vi "FollowAttackerTactic.vi"(8 "error in (no error)":errorcluster, 9 "Game in":refnum<class "Game.lvclass">, 10 "Robot":refnum<class "Robot.lvclass">, 11 "FollowAttackerTactic in":refnum<class "FollowAttackerTactic.lvclass">) -> (0 "error out":errorcluster, 2 "Robot out":refnum<class "Robot.lvclass">, 3 "FollowAttackerTactic out":refnum<class "FollowAttackerTactic.lvclass">)   [LabVIEW 2018, in "FollowAttackerTactic.lvclass"]
uses:
  FollowAttackerTactic.lvclass
  C:/Users/nicolas.oliveira/roboime/SSL_AI/Tactic_class/Tactic.lvclass
  Game_class/Game.lvclass
  Robot_class/Robot.lvclass
  Tactic_class/Tactic.lvclass/Tactic.ctl
  Skillbook_class/Skillbook.lvclass/Skillbook.ctl
  FollowAttackerTactic.lvclass/FollowAttackerTactic.ctl
  Skillbook_class/Read FollowAttackerSkill.lvclass.vi
  Tactic_class/Read Skillbook.vi
  Write States.vi
  Skillbook_class/Skillbook.lvclass
  FollowAttackerSkill_class/FollowAttackerSkill.lvclass
panel:
  out "x .or. y?":bool
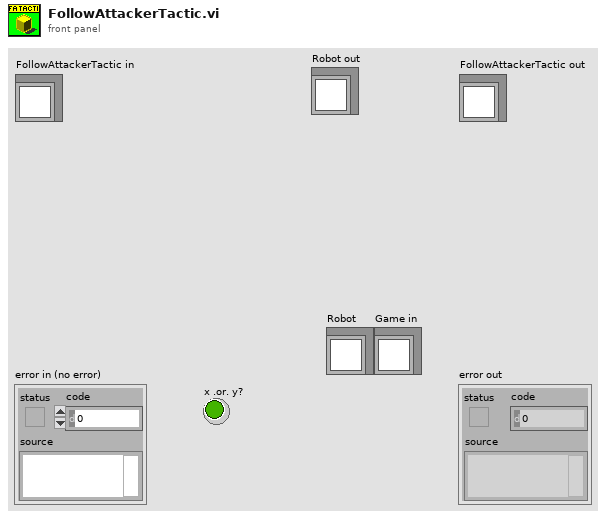
[diagram p1: front panel]
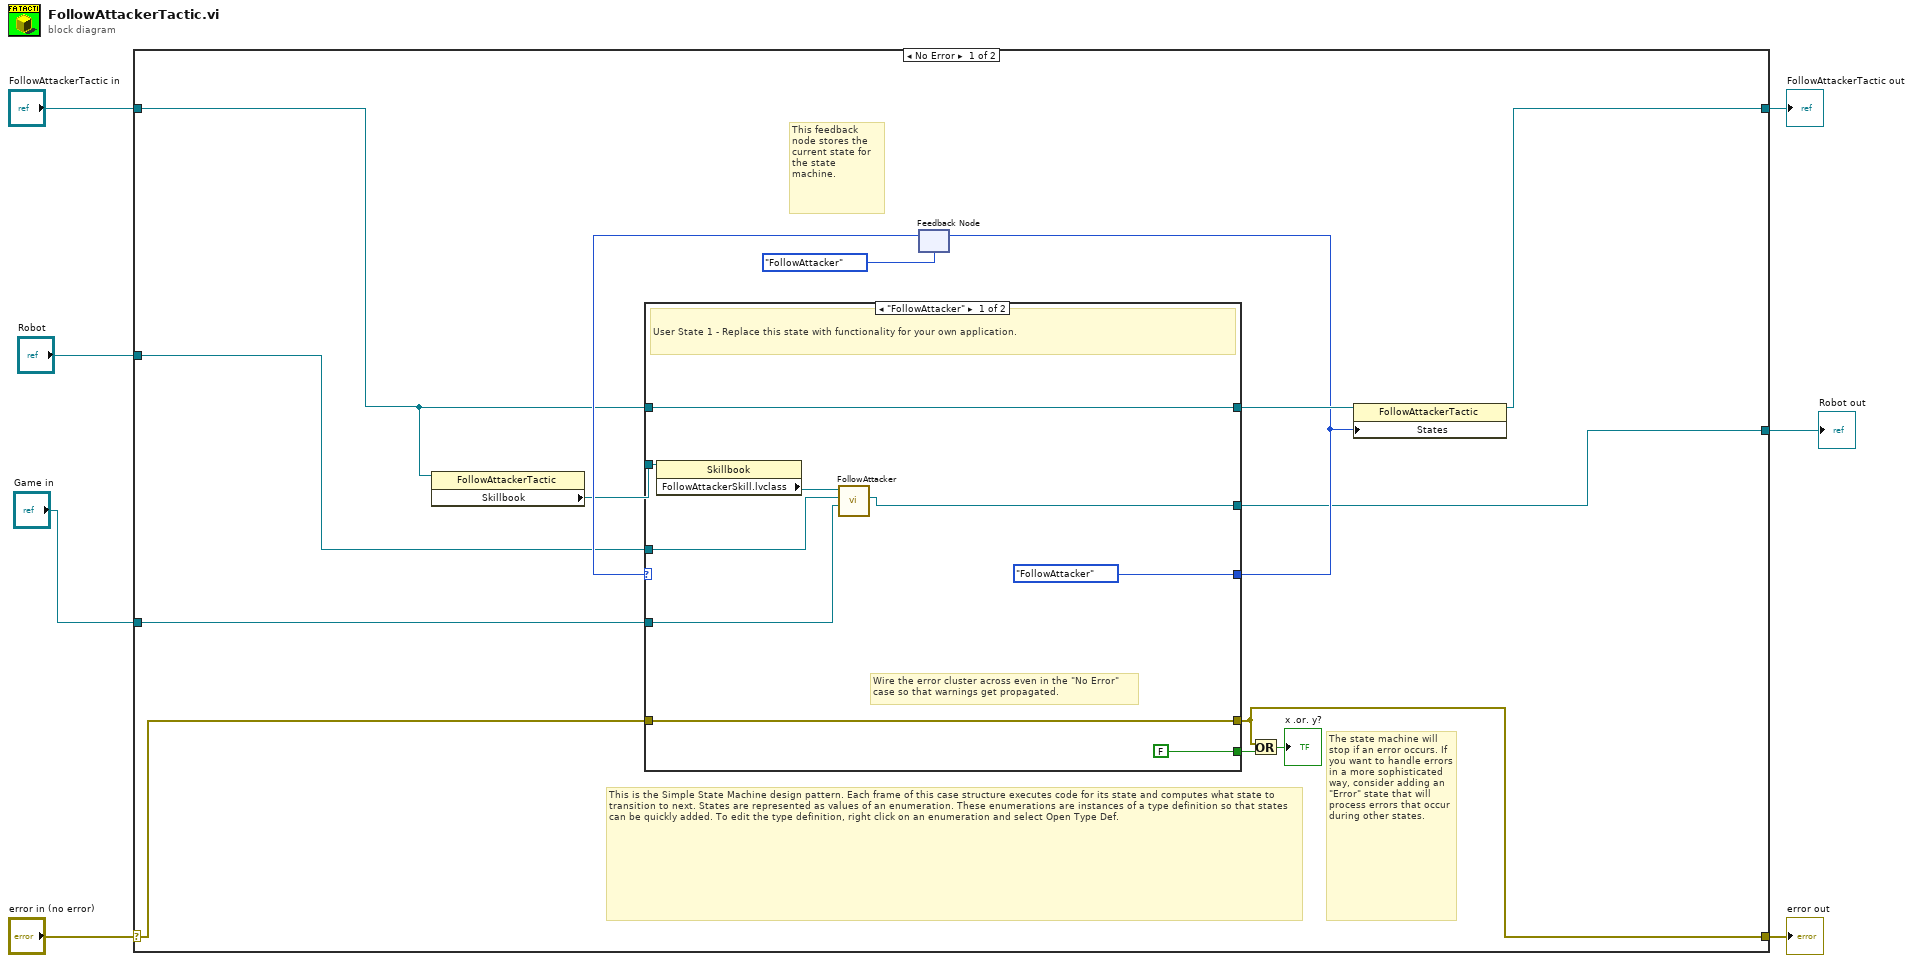
[diagram p0: block diagram]
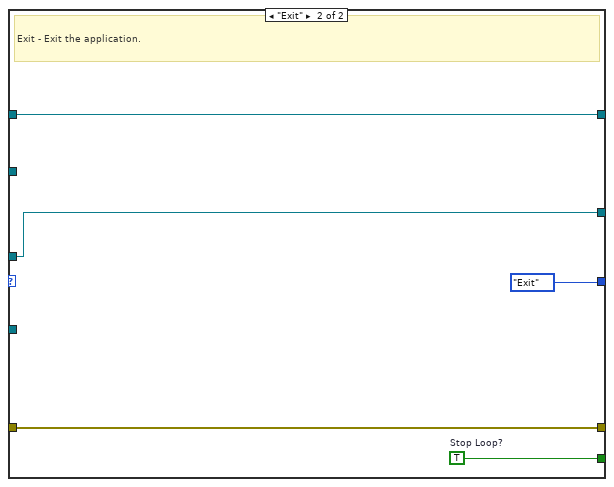
[diagram p2: hidden frame]
diagram:
  n1 = case shown="No Error" "error in (no error)" {
    selector: "error in (no error)" -> [w15 w38]
    tunnel: [w14 w38] -> w6
    tunnel: [w8 w37] -> w4
    tunnel: "FollowAttackerTactic in" -> [w13 w37]
    tunnel: "Robot" -> [w12 w36]
    tunnel: "Game in" -> [w11 _]
    tunnel: [w10 w36] -> w1
    frame No Error {
      # "The state machine will stop if an error occurs. If you want to handle errors in a more sophisticated way, consider adding an \"Error\" state that will process errors that occur during other states."
      # "This feedback node stores the current state for the state machine."
      # "This is the Simple State Machine design pattern. Each frame of this case structure executes code for its state and computes what state to transition to next. States are represented as values of an enumeration. These enumerations are instances of a type definition so that states can be quickly added. To edit the type definition, right click on an enumeration and select Open Type Def."
      # "Wire the error cluster across even in the \"No Error\"\ncase so that warnings get propagated."
      n2 = property class="FollowAttackerTactic"(reference=w13) -> ("Skillbook"=w18:refnum<class "Skillbook.lvclass">)  [unwired: 1 in, 2 out]
      n3 = feedback #1(enum16{"Exit", "FollowAttacker"}."FollowAttacker" ("States")) -> (w19:enum16{"Exit", "FollowAttacker"})
      n4 = case shown="\"FollowAttacker\"" w19 {
        tunnel: [enum16{"Exit", "FollowAttacker"}."FollowAttacker" ("States") enum16{"Exit", "FollowAttacker"}."Exit" ("States")] -> w16
        tunnel: [FALSE ("Stop Loop?") w35] -> w21
        tunnel: w15 -> [w29 w34]
        tunnel: [w29 w34] -> w14
        tunnel: w18 -> [w28 _]
        tunnel: w12 -> [w25 w33]
        tunnel: [w23 w33] -> w10
        tunnel: [w27 w32] -> w17
        tunnel: w13 -> [w27 w32]
        tunnel: w11 -> [w24 _]
        frame "FollowAttacker" {
          # "User State 1 - Replace this state with functionality for your own application."
          n5 = property class="Skillbook"(reference=w28) -> ("FollowAttackerSkill.lvclass"=w26:refnum<class "FollowAttackerSkill.lvclass">)  [unwired: 1 in, 2 out]
          n6 = call-dynamic "FollowAttacker.vi"("Game"=w24, "Robot"=w25, "FollowAttackerSkill in"=w26) -> ("Robot out"=w23:refnum<class "Robot.lvclass">)  [unwired: 6 in, 2 out]
        }
        frame "Exit" {
          w35 = TRUE  # Stop Loop?
          # "Exit - Exit the application."
        }
      }
      n7 = feedback-in #1(w16) -> ()
      n8 = Or(x=w14, y=w21) -> (x .or. y?=→"x .or. y?":bool)
      n9 = property class="FollowAttackerTactic"(reference=w17, "States"=w16) -> (reference out=w8:refnum<class "FollowAttackerTactic.lvclass">)  [unwired: 1 in, 1 out]
    }
    frame Error {
    }
  }
  "error out" <- w6
  "FollowAttackerTactic out" <- w4
  "Robot out" <- w1
